vi "Create.vi"() -> (0 "Connection":refnum<class "Connection.lvclass">)   [LabVIEW 2020, in "Connection.lvclass"]
uses:
  Connection.lvclass
  Connection.lvclass/Connection.ctl
  Element.ctl
  Tag Data.ctl
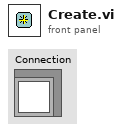
[diagram p1: front panel]
types:
  T1 = typedef "Connection.lvclass/Tag Data.ctl" = cluster{"Value":T2, "Updated":timestamp, "Sequence":u32}
  T2 = typedef "Connection.lvclass/Element.ctl" = dbl
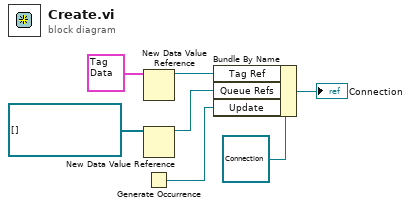
[diagram p0: block diagram]
diagram:
  n1 = New Data Value Reference(data value=T1 {"Value"=0.0, "Updated"=timestamp(0 s since 1904-01-01), "Sequence"=0} ("Tag Info")) -> (data value reference=w3:refnum<data-value>)  [unwired: 1 in, 1 out]
  n2 = New Data Value Reference(data value=refnum<queue>[] [] ("appended array")) -> (data value reference=w2:refnum<data-value>)  [unwired: 1 in, 1 out]
  n3 = Generate Occurrence() -> (w1:refnum<k4>)
  n4 = Bundle By Name(cluster=refnum<class "Connection.lvclass"> refnum ("Connection"), "Tag Ref"=w3, "Queue Refs"=w2, "Update"=w1) -> (→"Connection":refnum<class "Connection.lvclass">)
